vi "ROI_positions_SAVE.vi"(2 "Choice":string, 3 "XY positions":dbl[][](array[numeric]), 4 "error in":errorcluster, 7 "ROI LstBox Refnum":refnum<vi>) -> (0 "error out":errorcluster, 1 "XY positions OUT":dbl[][](array[numeric]))   [LabVIEW 2015]
uses:
  GLOBAL/Global_MAIN.vi
  GLOBAL/Global_ASI_stage.vi
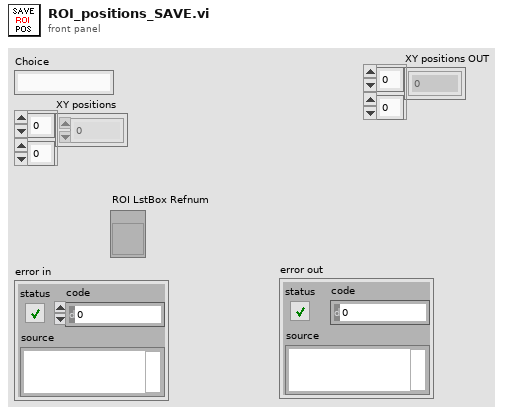
[diagram p1: front panel]
types:
  T1 = enum16{"open", "open or create", "create or replace", "create", "open (read-only)"}
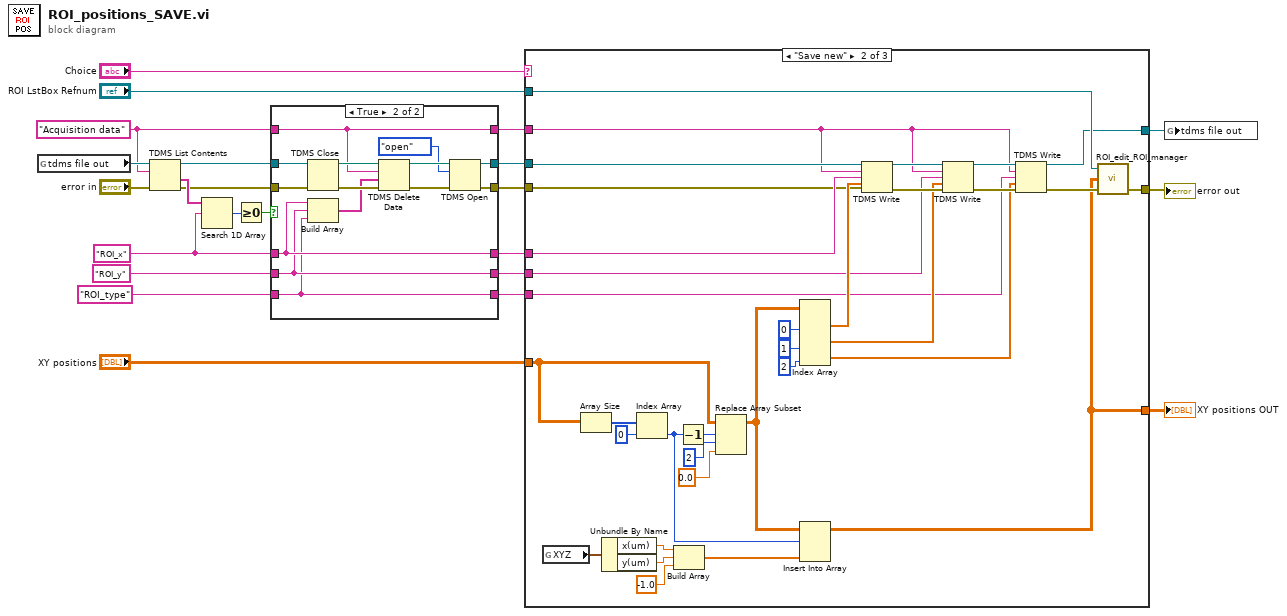
[diagram p0: block diagram]
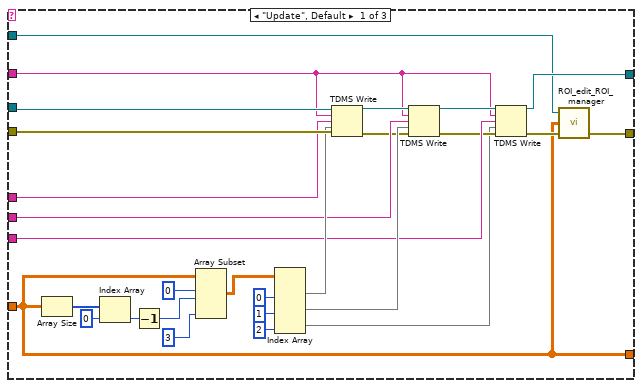
[diagram p3: hidden frame]
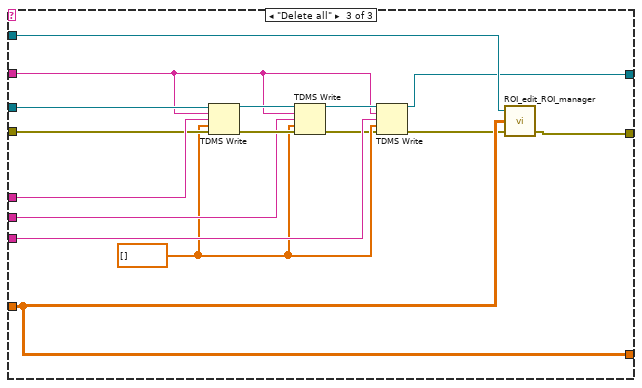
[diagram p4: hidden frame]
diagram:
  w9 = "ROI_x"
  w10 = "Acquisition data" ("group name in (Untitled)")
  n1 = global read "Global_MAIN.vi" "tdms file out"() -> (w13:refnum<k34>)
  n2 = TDMS List Contents(4:"error in", 6:w10, 7:w13) -> (0:w8:errorcluster, 1:w14:string[], 3:w11:refnum<k34>)  [unwired: 1 out]
  n3 = Search 1D Array(1D array=w14, element=w9) -> (index of element=w15:i32)  [unwired: 1 in]
  n4 = Greater Or Equal To 0?(x=w15) -> (x >= 0?=w7:bool)
  n5 = case shown="True" w7 {
    tunnel: "ROI_y" -> [w26 w32]
    tunnel: [w29 w37] -> w18
    tunnel: [w28 w36] -> w17
    tunnel: w11 -> [w29 w35]
    tunnel: w10 -> [w25 w31]
    tunnel: w9 -> [w27 w33]
    tunnel: w8 -> [w28 w34]
    tunnel: [w27 w33] -> w6
    tunnel: [w26 w32] -> w5
    tunnel: [w25 w31] -> w4
    tunnel: "ROI_type" -> [w24 w30]
    tunnel: [w24 w30] -> w2
    frame False {
    }
    frame True {
      n6 = TDMS Close(8:w34, 11:w35) -> (0:w42:errorcluster, 3:w43:path)
      n7 = Build Array(w33, w32, w30) -> (w41:string[])
      n8 = TDMS Delete Data(8:w42, 9:w41, 10:w31, 11:w43) -> (0:w39:errorcluster, 3:w40:path)  [unwired: 3 in]
      n9 = TDMS Open(8:w39, 10:T1."open" ("operation (0:open)"), 11:w40) -> (0:w36:errorcluster, 3:w37:refnum<k34>)  [unwired: 4 in]
    }
  }
  n10 = case shown="\"Save new\"" "Choice" {
    tunnel: [w46 w105 w121] -> w23
    tunnel: "XY positions" -> [w45 w75 w118]
    tunnel: [w45 w72 w118] -> w21
    tunnel: "ROI LstBox Refnum" -> [w44 w104 w120]
    tunnel: w4 -> [w51 w90 w111]
    tunnel: w6 -> [w63 w102 w119]
    tunnel: [w52 w89 w106] -> w16
    tunnel: w17 -> [w64 w95 w114]
    tunnel: w18 -> [w65 w94 w113]
    tunnel: w5 -> [w57 w99 w115]
    tunnel: w2 -> [w50 w87 w110]
    frame "Update", Default {
      n11 = Array Size(array=w45) -> (size(s)=w71:i32[])
      n12 = Index Array(array=w71, index=0) -> (element=w68:i32)
      n13 = Decrement(x=w68) -> (x-1=w67:i32)
      n14 = Array Subset(array=w45, index (row)=0 ("index"), length (row)=w67, length (col)=3 ("length")) -> (w62:dbl[][])  [unwired: 1 in]
      n15 = Index Array(array=w62, index (col) #1=0 ("disabled index (col)"), index (col) #2=1 ("index (col)"), index (col) #3=2 ("index (col)")) -> (element #1=w59:dbl[], element #2=w56:dbl[], element #3=w48:dbl[])  [unwired: 3 in]
      n16 = TDMS Write(0:w65, 5:w51, 7:w63, 9:w59, 11:w64) -> (4:w58:refnum<k34>, 15:w55:errorcluster)  [unwired: 1 in, 2 out]
      n17 = TDMS Write(0:w58, 5:w51, 7:w57, 9:w56, 11:w55) -> (4:w53:refnum<k34>, 15:w49:errorcluster)  [unwired: 1 in, 2 out]
      n18 = TDMS Write(0:w53, 5:w51, 7:w50, 9:w48, 11:w49) -> (4:w52:refnum<k34>, 15:w47:errorcluster)  [unwired: 1 in, 2 out]
      n19 = call "ROI_edit_ROI_manager.vi"("error in"=w47, "XY positions"=w45, "ROI Refnum"=w44) -> ("error out"=w46:errorcluster)  [unwired: 2 in]
    }
    frame "Save new" {
      n20 = global read "Global_ASI_stage.vi" "XYZ"() -> (w80:cluster{"x(um)":dbl, "y(um)":dbl, "z(um)":dbl})
      n21 = Array Size(array=w75) -> (size(s)=w81:i32[])
      n22 = Unbundle By Name(w80) -> ("x(um)"=w79:dbl, "y(um)"=w78:dbl)
      n23 = Index Array(array=w81, index=0) -> (element=w76:i32)
      n24 = Build Array(w79, w78, -1.0 ("element")) -> (w83:dbl[])
      n25 = Decrement(x=w76) -> (x-1=w74:i32)
      n26 = Replace Array Subset(array=w75, new element=0.0 ("new element/subarray"), index (row)=w74, index (col)=2 ("disabled index (col)")) -> (w73:dbl[][])
      n27 = Index Array(array=w73, index (col) #1=0 ("disabled index (col)"), index (col) #2=1 ("index (col)"), index (col) #3=2 ("index (col)")) -> (element #1=w101:dbl[], element #2=w97:dbl[], element #3=w88:dbl[])  [unwired: 3 in]
      n28 = Insert Into Array(array=w73, index (row)=w76, new element=w83) -> (w72:dbl[][])  [unwired: 1 in]
      n29 = TDMS Write(0:w94, 5:w90, 7:w102, 9:w101, 11:w95) -> (4:w96:refnum<k34>, 15:w100:errorcluster)  [unwired: 1 in, 2 out]
      n30 = TDMS Write(0:w96, 5:w90, 7:w99, 9:w97, 11:w100) -> (4:w92:refnum<k34>, 15:w91:errorcluster)  [unwired: 1 in, 2 out]
      n31 = TDMS Write(0:w92, 5:w90, 7:w87, 9:w88, 11:w91) -> (4:w89:refnum<k34>, 15:w86:errorcluster)  [unwired: 1 in, 2 out]
      n32 = call "ROI_edit_ROI_manager.vi"("error in"=w86, "XY positions"=w72, "ROI Refnum"=w104) -> ("error out"=w105:errorcluster)  [unwired: 2 in]
    }
    frame "Delete all" {
      w109 = dbl[] [] ("subarray")
      n33 = TDMS Write(0:w113, 5:w111, 7:w119, 9:w109, 11:w114) -> (4:w117:refnum<k34>, 15:w116:errorcluster)  [unwired: 1 in, 2 out]
      n34 = TDMS Write(0:w117, 5:w111, 7:w115, 9:w109, 11:w116) -> (4:w112:refnum<k34>, 15:w108:errorcluster)  [unwired: 1 in, 2 out]
      n35 = TDMS Write(0:w112, 5:w111, 7:w110, 9:w109, 11:w108) -> (4:w106:refnum<k34>, 15:w107:errorcluster)  [unwired: 1 in, 2 out]
      n36 = call "ROI_edit_ROI_manager.vi"("error in"=w107, "XY positions"=w118, "ROI Refnum"=w120) -> ("error out"=w121:errorcluster)  [unwired: 2 in]
    }
  }
  "error out" <- w23
  "XY positions OUT" <- w21
  n37 = global write "Global_MAIN.vi" "tdms file out"(w16) -> ()
